vi "GlobalVariant.vi"() -> ()   [LabVIEW 2023]
panel:
  in  "SystemRunFlag":u16
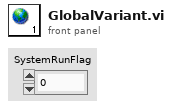
[diagram p1: front panel]
diagram:
